vi "Configure Memory.vi"(0 "VISA resource name":refnum<visa-resource-name>, 5 "Memory (1)":i32=1 min=1 max=50 step=1, 7 "Memory Cycle (1)":i32=1 min=0 max=9999 step=1, 11 "error in (no error)":errorcluster) -> (4 "VISA resource name out":refnum<visa-resource-name>, 15 "error out":errorcluster)   [LabVIEW 2016, in "APT 300XAC Series.lvlib"]
doc: "Configures memory and memory cycle in the power source instrument.\n\nThe instrument has 50 memory locations within it. Each memory can be programmed one at a time. There are 9 steps in every memory.\nThe memory cycle represents the number of times the test is to be repeated on the particular memory location."
uses:
  APT 300XAC Series.lvlib
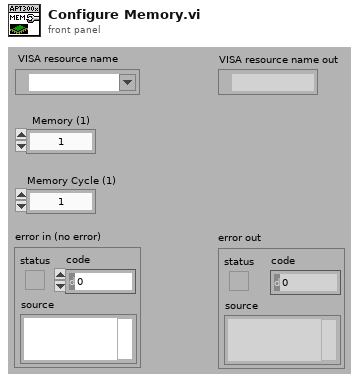
[diagram p1: front panel]
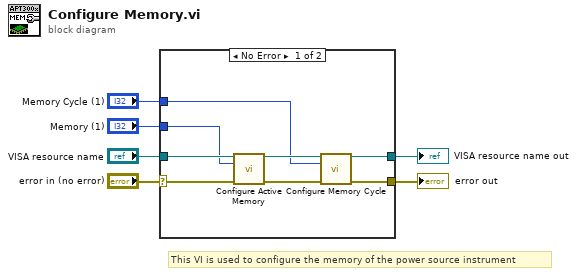
[diagram p0: block diagram]
diagram:
  # "This VI is used to configure the memory of the power source instrument"
  n1 = case shown="No Error" "error in (no error)" {
    selector: "error in (no error)" -> [w9 w15]
    tunnel: [w14 w15] -> w6
    tunnel: [w13 w16] -> w5
    tunnel: "VISA resource name" -> [w12 w16]
    tunnel: "Memory (1)" -> [w8 _]
    tunnel: "Memory Cycle (1)" -> [w7 _]
    frame No Error {
      n2 = call "Configure Active Memory.vi"("VISA resource name"=w12, "Memory (1)"=w8, "error in (no error)"=w9) -> ("VISA resource name out"=w10:refnum<visa-resource-name>, "error out"=w11:errorcluster)  [unwired: 11 in]
      n3 = call "Configure Memory Cycle.vi"("VISA resource name"=w10, "Memory Cycle (1)"=w7, "error in (no error)"=w11) -> ("VISA resource name out"=w13:refnum<visa-resource-name>, "error out"=w14:errorcluster)  [unwired: 11 in]
    }
    frame Error {
    }
  }
  "error out" <- w6
  "VISA resource name out" <- w5
